vi "Get Run Remote Services.vi"(8 "error in (no error)":errorcluster, 11 "Vecto in":refnum<class "Vecto.lvclass">) -> (0 "error out":errorcluster, 2 "Run Remote Services":bool, 3 "Vecto out":refnum<class "Vecto.lvclass">)   [LabVIEW 2020, in "Vecto.lvlib" / "Vecto.lvclass"]
uses:
  Vecto.lvclass
  Vecto.lvclass/Vecto.ctl
  Node Config/Node Config.lvclass
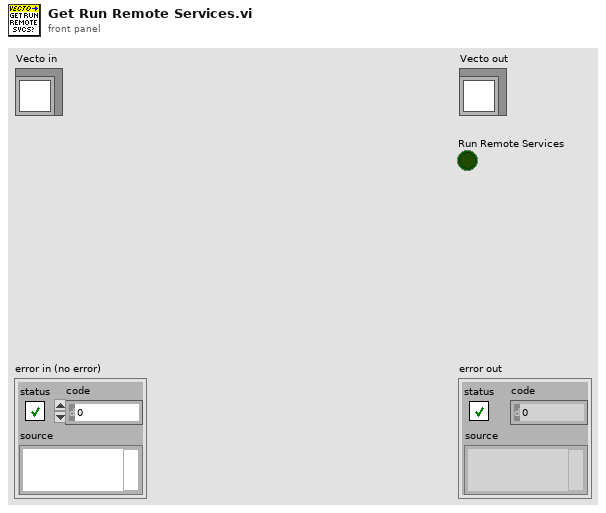
[diagram p1: front panel]
types:
  T1 = typedef "Vecto.lvlib/Comms Features.ctl" = cluster{"HTTP Server":bool, "TCP Messaging":bool, "Remote Data":bool, "Discovery":bool}
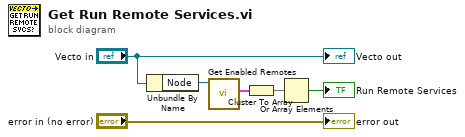
[diagram p0: block diagram]
diagram:
  n1 = Unbundle By Name("Vecto in") -> ("Node"=w4:refnum<class "Node Config.lvclass">)
  n2 = call "Get Enabled Remotes.vi"("Node Config in"=w4) -> ("Comms Features"=w3:T1)  [unwired: 8 in, 2 out]
  n3 = Cluster To Array(cluster=w3) -> (array=w2:bool[])
  n4 = Or Array Elements(Boolean array=w2) -> (logical OR=→"Run Remote Services":bool)
  "error out" <- "error in (no error)"
  "Vecto out" <- "Vecto in"
